vi "LUTQuery.vi"() -> ()   [LabVIEW 2020, in "ORM_Examples.lvlib"]
uses:
  ORM_Examples.lvlib
  <vilib>/Viviota/shared/ORM_lib.lvlibp/ObjectRow/ObjectLUT.lvclass
  <vilib>/Viviota/shared/ORM.lvlibp/ORM/TypeMap/TypeMap.lvclass
  d1c1baa4-be1d-406a-bc71-ac5b39482f5d.vi
  d1c1baa4-be1d-406a-bc71-ac5b39482f5d.vi/a9ccc3c9-891a-4d80-8d4f-837bdef88ccd.vi
  d1c1baa4-be1d-406a-bc71-ac5b39482f5d.vi/8216614f-f413-45b3-8111-14f8d0271ea5.vi
  d1c1baa4-be1d-406a-bc71-ac5b39482f5d.vi/fc6a5c23-d21f-4d2c-895e-66da96fa9491.vi
  d1c1baa4-be1d-406a-bc71-ac5b39482f5d.vi/fc6a5c23-d21f-4d2c-895e-66da96fa9491.vi/9d007ba8-e96f-4737-8d8a-6b46cf7f5c4a.vi
  d1c1baa4-be1d-406a-bc71-ac5b39482f5d.vi/fc6a5c23-d21f-4d2c-895e-66da96fa9491.vi/050765a8-e5d4-4415-b637-62775228e838.vi
  <vilib>/Viviota/shared/ORM_ADONet.lvlibp/ADOMapper/ADOMapper.lvclass
  C:/Program Files/National Instruments/LabVIEW 2024/vi.lib/Viviota/shared/ORM.lvlibp/ORM/SqlMapper/SqlMapper.lvclass
  <vilib>/Viviota/shared/ORM.lvlibp/ORM/TypeMap/Write Table Name.vi
  <vilib>/Viviota/shared/ORM.lvlibp/ORM/TypeMap/Write Autokey.vi
  <vilib>/Viviota/shared/ORM_lib.lvlibp/ObjectRow/Write LUT.vi
  <vilib>/Viviota/shared/ORM_DBC_Sqlite.lvlibp/Sqlite Connect.vi
  <vilib>/Utility/error.llb/Error Cluster From Error Code.vi
  <vilib>/Viviota/shared/ORM.lvlibp/ORM/TypeMap/Read TypeMap.vi
  <vilib>/Viviota/shared/ORM.lvlibp/ORM/TypeMap/Where.vi
  <vilib>/Viviota/shared/ORM.lvlibp/ORM/Query Result/Next.vi
  <vilib>/Viviota/shared/ORM.lvlibp/ORM/TypeMap/ToLabVIEW_Wrap.vi
  <vilib>/Viviota/shared/ORM.lvlibp/ORM/SqlMapper/End Transaction.vi
  <vilib>/Viviota/shared/ORM_lib.lvlibp/ObjectRow/Read LUT.vi
  <vilib>/Viviota/shared/ORM.lvlibp/ORM/Query Result/Query Result.lvclass
  ORM_API/ORM_API.lvlib
  <vilib>/Viviota/shared/ORM_ADONet.lvlibp
  <vilib>/Viviota/shared/ORM_DBC_Sqlite.lvlibp/DBC.lvclass
  C:/Program Files/National Instruments/LabVIEW 2024/vi.lib/Viviota/shared/ORM_ADONet.lvlibp/ADOMapper/ADOMapper.lvclass
panel:
  out "Array":variant[](array[variant])
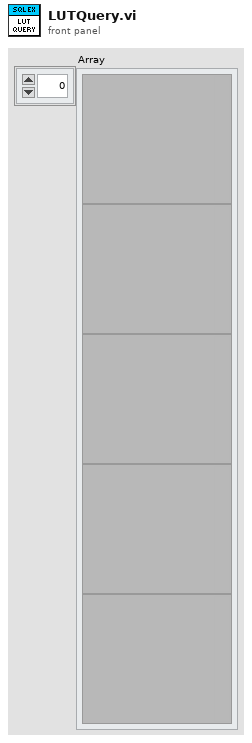
[diagram p1: front panel]
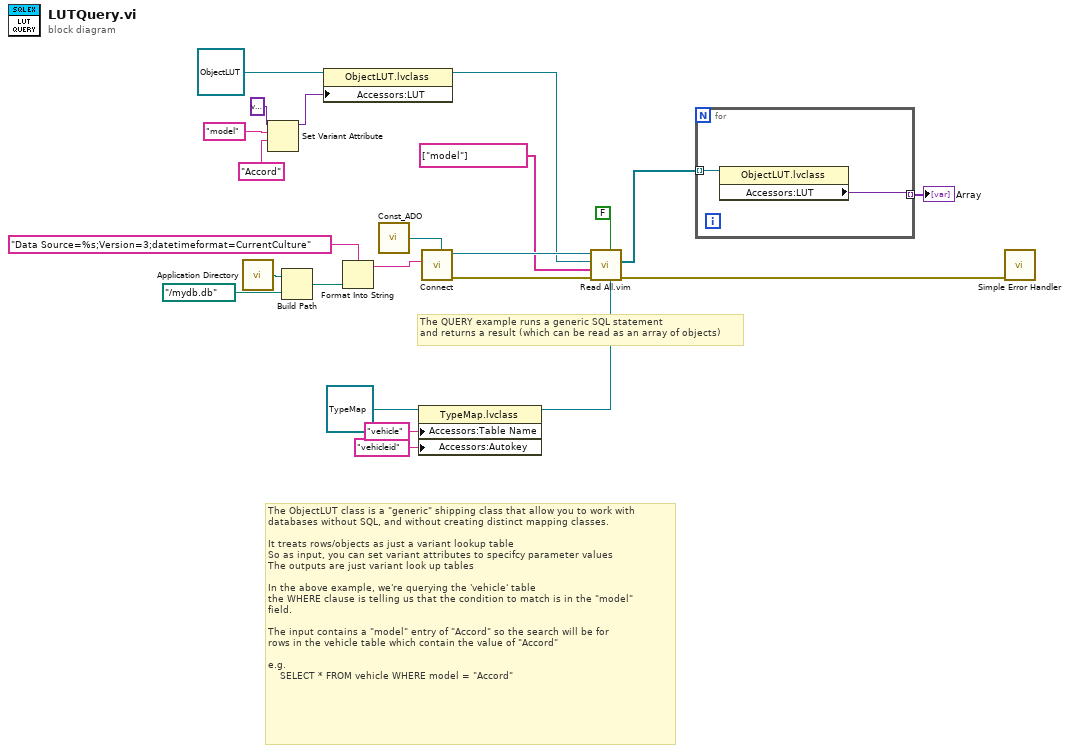
[diagram p0: block diagram]
diagram:
  # "The ObjectLUT class is a \"generic\" shipping class that allow you to work with \ndatabases without SQL, and without creating distinct mapping classes.\n\nIt treats rows/objects as just a variant lookup table\nSo as input, you can set variant attributes to specifcy parameter values\nThe outputs are just variant look up tables\n\nIn the above example, we're querying the 'vehicle' table\nthe WHERE clause is telling us that the condition to match is in the \"model\"\nfield.\n\nThe input contains a \"model\" entry of \"Accord\" so the search will be for \nrows in the vehicle table which contain the value of \"Accord\"\n\ne.g. \n    SELECT * FROM vehicle WHERE model = \"Accord\""
  # "The QUERY example runs a generic SQL statement\nand returns a result (which can be read as an array of objects)"
  n1 = call <vilib>:"Application Directory.vi"() -> ("Application Directory"=w22:path)
  n2 = Set Variant Attribute(Variant=variant ("variant"), name="model", value="Accord" ("name")) -> (Variant out=w5:variant)  [unwired: 1 in, 2 out]
  n3 = Build Path(base path=w22, name or relative path=path "../mydb.db" ("file out")) -> (appended path=w23:path)
  n4 = property class="ObjectLUT.lvclass"(reference=refnum<class "ObjectLUT.lvclass"> refnum ("ORM_lib.lvlibp:ObjectLUT.lvclass"), "Accessors:LUT"=w5) -> (reference out=w6:refnum<class "ObjectLUT.lvclass">)  [unwired: 1 in, 1 out]
  n5 = Format Into String(format string="Data Source=%s;Version=3;datetimeformat=CurrentCulture" ("connectionStringName"), w23) -> (resulting string=w18:string)  [unwired: 2 in, 1 out]
  n6 = call <vilib>:"Const_ADO.vi"() -> ("ADOMapper"=w19:refnum<class "ADOMapper.lvclass">)
  n7 = property class="TypeMap.lvclass"(reference=refnum<class "TypeMap.lvclass"> refnum ("TypeMap in"), "Accessors:Table Name"="vehicle" ("Table Name"), "Accessors:Autokey"="vehicleid" ("Autokey")) -> (reference out=w12:refnum<class "TypeMap.lvclass">)  [unwired: 1 in, 1 out]
  n8 = call-poly "Connect.vi"("SqlMapper Type"=w19, "Connection String"=w18) -> ("error out"=w17:errorcluster, "SqlMapper out"=w16:refnum<class "ADOMapper.lvclass">)  [unwired: 8 in]
  n9 = call "Read All.vim"("TypeMap in"=w12, "Select All"=FALSE, "error in (no error)"=w17, "WHERE"=string[] ["model"], "Object"=w6, "SqlMapper in"=w16) -> ("error out"=w15:errorcluster, "Query Results"=w9:refnum<class "ObjectLUT.lvclass">[])  [unwired: 3 in, 1 out]
  n10 = for {
    tunnel: w9 -> [w25] mode=indexing
    tunnel: [w24] -> w8 mode=indexing
    n11 = property class="ObjectLUT.lvclass"(reference=w25) -> ("Accessors:LUT"=w24:variant)  [unwired: 1 in, 2 out]
  }
  "Array" <- w8
  n12 = call <vilib>:"Simple Error Handler.vi"("error in (no error)"=w15) -> ()  [unwired: 4 in, 5 out]
